vi "NI6071E.evt call get DAQ Status.vi"(0 "i ref in":refnum<vi>, 2 "Client":string, 3 "Client timeout (10000)":i32=10000, 5 "error in":errorcluster) -> (14 "i ref out":refnum<vi>, 16 "err unpacking data":bool, 17 "Client Status":string, 19 "error out":errorcluster)   [LabVIEW 2014, in "NI6071E.lvlib"]
doc: "This VI asks for an event by a synchronous call"
uses:
  NI6071E.lvlib
  NI6071ECommand.ctl
  CSCore/CSSystem/CoreLib/CoreLib.byte array 2 string.vi
  CSCore/CSSystem/CoreLib/CoreLib.int 2 byte array.vi
  CSCore/BaseProcess/BaseProcess.lvlib
  CSCore/CSSystem/CoreLib/CoreLib.lvlib
panel:
  in  "NI6071E Command":T1=enum."GetDAQStatus"
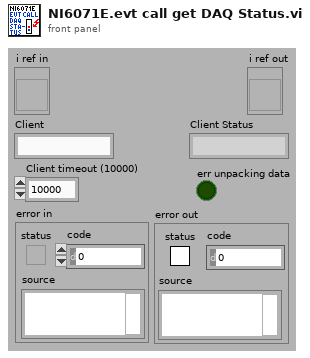
[diagram p1: front panel]
types:
  T1 = typedef "NI6071E.lvlib/NI6071ECommand.ctl" = enum16{"Ping", "Reset", "ConfigureDAQ", "StartDAQ", "StopDAQ", "GetDAQStatus", "ReadData", "SaveData", "CloseConnection"}
  T2 = enum16{"simple", "synchronous", "asynchronous", "notification"}
  T3 = typedef "CoreDefs.rawDataType.ctl" = i8[]
  T4 = typedef "CoreDefs.call_type.ctl" = cluster{"Object":string, "Selector":string, "CallType":enum16{"simple", "synchronous", "asynchronous"}, "Async Object":string, "Async Selector":string, "Data Descriptor":T5, "Data":T3, "Error #":i32, "Expire":u32}
  T5 = typedef "BaseProcess.lvlib/BaseProcess.descriptor string definition.ctl" = string
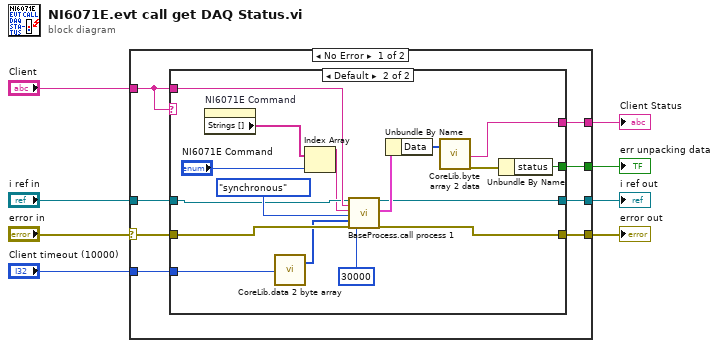
[diagram p0: block diagram]
diagram:
  n1 = case shown="No Error" "error in" {
    selector: "error in" -> [w11 w36]
    tunnel: "Client timeout (10000)" -> [w10 _]
    tunnel: [w16 w36] -> w7
    tunnel: "i ref in" -> [w15 w37]
    tunnel: "Client" -> [w9 _]
    tunnel: [w14 w37] -> w4
    tunnel: [w13 _] -> w3
    tunnel: [w12 _] -> w2
    frame No Error {
      n2 = case shown="Default" w9 {
        tunnel: [w17 w34] -> w16
        tunnel: w15 -> [w18 w23]
        tunnel: w9 -> [_ w32]
        tunnel: [w18 w22] -> w14
        tunnel: [_ w29] -> w13
        tunnel: [_ w27] -> w12
        tunnel: w11 -> [w17 w26]
        tunnel: w10 -> [_ w25]
        frame "N/A" {
        }
        frame Default {
          n3 = property on="NI6071E Command" class="Enum (strict)"() -> ("Strings []"=w19:string[])  [unwired: 2 in, 2 out]
          n4 = call-poly "CoreLib.data 2 byte array.vi"("i32"=w25) -> ("byteArray out"=w24:T3)  [unwired: 18 in]
          n5 = Index Array(array=w19, index="NI6071E Command") -> (element=w20:string)
          n6 = call "BaseProcess.call process 1.vi"("i ref in"=w23, "Object"=w32, "Selector"=w20, "CallType"=T2."synchronous", "Data"=w24, "error in (no error)"=w26, "timeout (ms)"=30000) -> ("i ref out"=w22:refnum<vi>, "call cluster out"=w35:T4, "error out"=w34:errorcluster)  [unwired: 10 in]
          n7 = Unbundle By Name(w35) -> ("Data"=w30:T3)
          n8 = call-poly "CoreLib.byte array 2 data.vi"("byteArray"=w30) -> ("string"=w29:string, "error out"=w28:errorcluster)  [unwired: 16 in, 1 out]
          n9 = Unbundle By Name(w28) -> ("status"=w27:bool)
        }
      }
    }
    frame Error {
    }
  }
  "Client Status" <- w3
  "error out" <- w7
  "i ref out" <- w4
  "err unpacking data" <- w2
